vi "dfd_FXP AntiSymmetric FIR with IS.vi"(6 "state in":i64[](array[numeric]), 7 "FXPOPs":T5[](array[typedef]) {"source" items=["Coef a/k"=0, "Coef b/v"=7, "Input"=1, "Output"=2, "Multiplicand"=3, "Product"=4, "Sum"=5, "Delay"=6, "Gain"=8]}, 8 "filtering statistics in":T4(array[cluster]) {"statistics information"."min value" format="%.2f"; "statistics information"."max value" format="%.2f"; "Quantizer Source" items=["Coefficients a/k"=0, "Coefficients b/v"=7, "Input"=1, "Output"=2, "Multiplicand"=3, "Product"=4, "Sum"=5, "Delay"=6]}, 10 "coef b":T7, 11 "X":T7) -> (0 "filtering statistics out":T4(array[cluster]) {"statistics information"."min value" format="%.2f"; "statistics information"."max value" format="%.2f"; "Quantizer Source" items=["Coefficients a/k"=0, "Coefficients b/v"=7, "Input"=1, "Output"=2, "Multiplicand"=3, "Product"=4, "Sum"=5, "Delay"=6]}, 3 "filtered X":T7, 4 "state out":i64[](array[numeric]))   [LabVIEW 2017, in "NI_DigFilter_FXP.lvlib"]
uses:
  <vilib>/addons/Digital Filter Design/NI_DigFilter_FXP.lvlib
  <vilib>/addons/Digital Filter Design/_Objects.llb/dfd_DFXP Data Type (vector).ctl
  <vilib>/addons/Digital Filter Design/_Objects.llb/dfd_DFXP Operation Parameter.ctl
  <vilib>/addons/Digital Filter Design/_Objects.llb/dfd_Internal Quantization Srcs.ctl
  <vilib>/addons/Digital Filter Design/_Objects.llb/DFD Quantization Sources.ctl
  <vilib>/addons/Digital Filter Design/_Objects.llb/DFD FXP Statistics Data.ctl
  <vilib>/addons/Digital Filter Design/_Objects.llb/dfd_DFXP Data Type (scaler).ctl
  <vilib>/addons/Digital Filter Design/NI_DigFilterLicensed.lvlib
panel:
  in  "DFXP Value":T1={"value"=0, "wl"=0, "iwl"=0, "Signed"=TRUE} {"value" format="%.0x"}
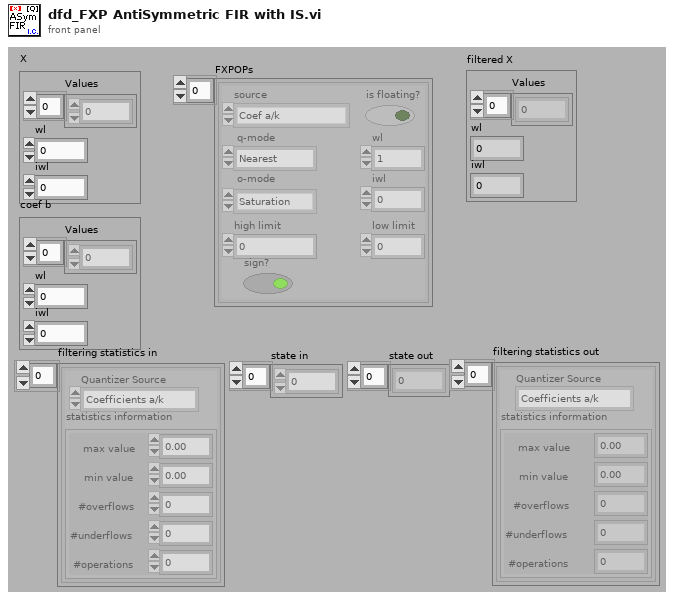
[diagram p1: front panel]
types:
  T1 = typedef "dfd_DFXP Data Type (scaler).ctl" = cluster{"value":i64, "wl":i16, "iwl":i16, "Signed":bool}
  T2 = typedef "NI_DigFilterLicensed.lvlib/DFD Quantization Sources.ctl" = u16
  T3 = typedef "NI_DigFilterLicensed.lvlib/DFD FXP Statistics Data.ctl" = cluster{"max value":ext, "min value":ext, "#overflows":i32, "#underflows":i32, "#operations":i32}
  T4 = cluster{"Quantizer Source":T2, "statistics information":T3}[]
  T5 = typedef "dfd_DFXP Operation Parameter.ctl" = cluster{"source":T6, "is floating?":bool, "o-mode":enum16{"Saturation", "Wrap"}, "q-mode":enum16{"Nearest", "Truncation"}, "wl":i16, "high limit":i64, "low limit":i64, "iwl":i16, "sign?":bool}
  T6 = typedef "NI_DigFilterLicensed.lvlib/dfd_Internal Quantization Srcs.ctl" = u16
  T7 = typedef "dfd_DFXP Data Type (vector).ctl" = cluster{"Values":i64[], "wl":i16, "iwl":i16}
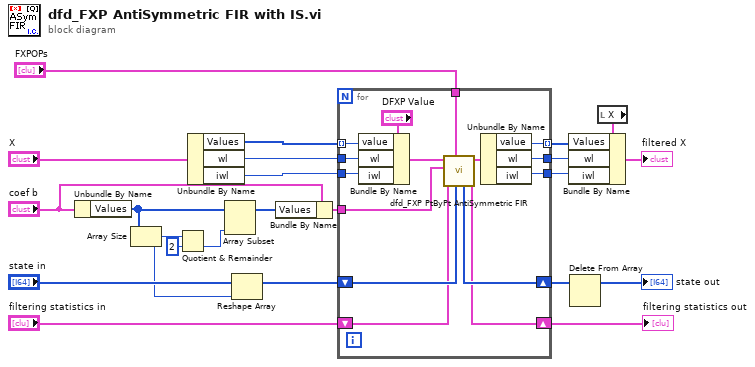
[diagram p0: block diagram]
diagram:
  n1 = Unbundle By Name("coef b") -> ("Values"=w10:i64[])
  n2 = Array Size(array=w10) -> (size(s)=w18:i32)
  n3 = Quotient & Remainder(x=w18, y=2) -> (floor(x/y)=w17:i32)  [unwired: 1 out]
  n4 = Unbundle By Name("X") -> ("Values"=w7:i64[], "wl"=w6:i16, "iwl"=w5:i16)
  n5 = Array Subset(array=w10, length=w17) -> (w20:i64[])  [unwired: 1 in]
  n6 = Reshape Array("state in", w18) -> (w21:i64[])
  n7 = Bundle By Name(cluster="coef b", "Values"=w20) -> (w9:T7)
  n8 = for {
    tunnel: w7 -> [w31] mode=indexing
    tunnel: w9 -> [w32]
    shift-right: [w36] -> w15
    shift-left: w21 -> [w37]
    tunnel: [w26] -> w16 mode=indexing
    tunnel: "FXPOPs" -> [w35]
    shift-right: [w33] -> w12
    shift-left: "filtering statistics in" -> [w34]
    tunnel: w6 -> [w28]
    tunnel: w5 -> [w27]
    tunnel: [w25] -> w2
    tunnel: [w24] -> w1
    n9 = Bundle By Name(cluster="DFXP Value", "value"=w31, "wl"=w28, "iwl"=w27) -> (w30:T1)
    n10 = call <vilib>:"dfd_FXP PtByPt AntiSymmetric FIR.vi"("state in"=w37, "FXPOPs"=w35, "filtering statistics in"=w34, "coef b (half storage)"=w32, "x"=w30) -> ("filtering statistics out"=w33:T4, "filtered x"=w38:T1, "state out"=w36:i64[])  [unwired: 4 out]
    n11 = Unbundle By Name(w38) -> ("value"=w26:i64, "wl"=w25:i16, "iwl"=w24:i16)
  }
  "filtering statistics out" <- w12
  n12 = Delete From Array(array=w15) -> (array with subset deleted=→"state out":i64[])  [unwired: 2 in, 1 out]
  n13 = local read "X"() -> (w3:T7)
  n14 = Bundle By Name(cluster=w3, "Values"=w16, "wl"=w2, "iwl"=w1) -> (→"filtered X":T7)
